vi "Test Error from Invalid Image.vi"(8 "error in (no error)":errorcluster, 11 "Test Case In":refnum<class "01_Image.lvclass">) -> (0 "error out":errorcluster, 3 "Test Case Out":refnum<class "01_Image.lvclass">)   [LabVIEW 2020, in "test.lvlib" / "01_Image.lvclass"]
uses:
  01_Image.lvclass
  C:/Program Files (x86)/National Instruments/LabVIEW 2020/vi.lib/Astemes/LUnit/Test Case.lvclass
  common/Image Size (Integer).ctl
  <vilib>/Astemes/LUnit/Test Case.lvclass/Test Case.ctl
  image/New Image (Greyscale Preallocated).vi
  image/New Image (Greyscale Preallocated).vi/6598b9e0-8a08-46f5-91fd-ca1b87217137.vi
  <vilib>/Astemes/LUnit/Append Fail Result.vi
  <vilib>/Astemes/LUnit/Append Pass Result.vi
  <vilib>/Astemes/LUnit/Run In UI.vi
  <vilib>/Utility/error.llb/Clear Errors.vi
  <vilib>/Utility/error.llb/Error Cluster From Error Code.vi
  image/image.lvlib
  <vilib>/Astemes/LUnit/Test Case.lvclass
  common/common.lvlib
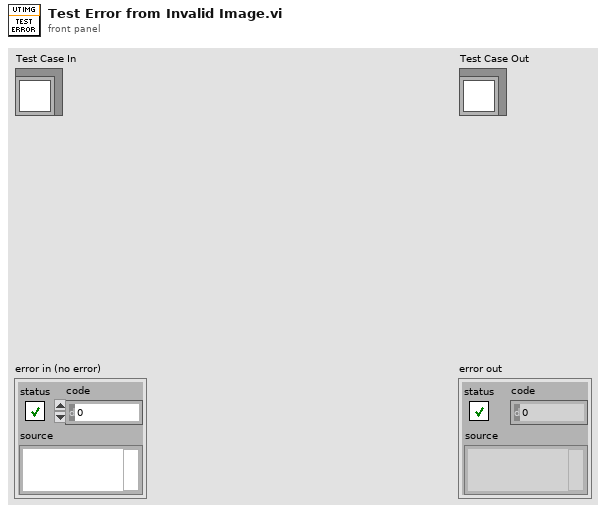
[diagram p1: front panel]
types:
  T1 = typedef "common.lvlib/Image Size (Integer).ctl" = cluster{"Width":u16, "Height":u16}
  T2 = typedef "image.lvlib/Greyscale Image.ctl" = refnum<data-value>
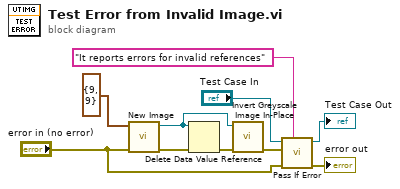
[diagram p0: block diagram]
diagram:
  n1 = call-poly "New Image.vi"("error in (no error)"="error in (no error)", "Preallocated Image Size (Default 0,0)"=T1 {"Width"=9, "Height"=9}) -> ("error out"=w7:errorcluster, "Greyscale Image"=w5:T2)  [unwired: 8 in]
  n2 = Delete Data Value Reference(data value reference=w5, error in=w7) -> (error out=w6:errorcluster)  [unwired: 1 out]
  n3 = call "Invert Greyscale Image In-Place.vi"("error in (no error)"=w6, "Greyscale Image to Invert in Place in"=w5) -> ("error out"=w4:errorcluster)  [unwired: 8 in, 1 out]
  n4 = call <vilib>:"Pass If Error.vi"("Description"="It reports errors for invalid references", "error in (no error)"="error in (no error)", "Assert error"=w4, "LUnit Test Case In"="Test Case In") -> ("error out"=→"error out":errorcluster, "LUnit Test Case Out"=→"Test Case Out":refnum<class "01_Image.lvclass">)  [unwired: 6 in]
